vi "FFRS.VI"   [LabVIEW 2015]
uses:
  lwlscdll.dll
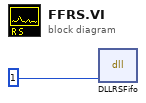
[diagram p0: block diagram]
diagram:
  n1 = dll-call lib="G:/SD/IR-det/lv/2cam/board.vis/lwlscdll.dll" fn="DLLRSFifo"("drv"=u32 1) -> ()  [unwired: 5 in, 2 out]
